vi "start panels.vi"(8 "error in":errorcluster) -> (0 "error out":errorcluster, 2 "vi names":string[](array[string]), 3 "vi refs":refnum<vi>[](array[refnum]))   [LabVIEW 2017]
panel:
  in  "visible":bool[](array[boolean])=[FALSE, FALSE, FALSE, FALSE, FALSE]
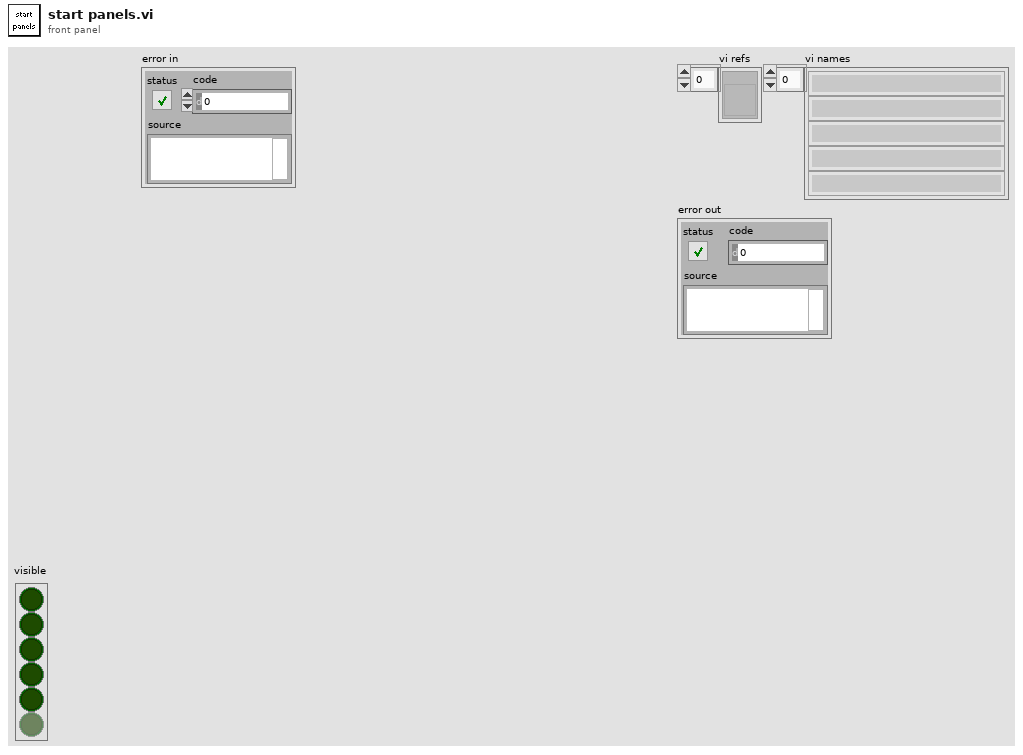
[diagram p1: front panel]
types:
  T1 = enum32{"Invalid", "Standard", "Closed", "Hidden", "Minimized", "Maximized"}
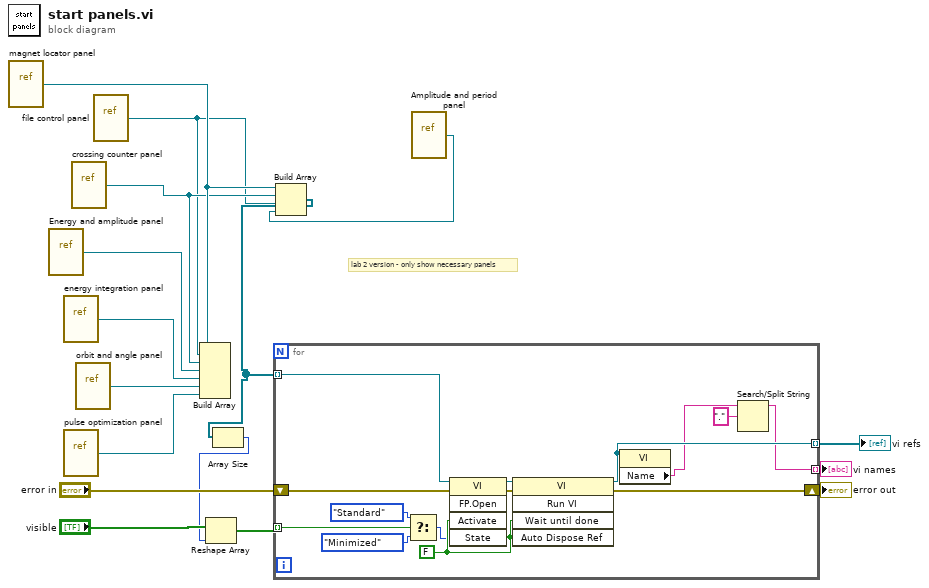
[diagram p0: block diagram]
diagram:
  # "lab 2 version - only show necessary panels"
  n1 = vi-ref "magnet locator panel.vi"() -> (w6:refnum<vi>)
  n2 = vi-ref "Energy and amplitude panel.vi"() -> (w15:refnum<vi>)
  n3 = vi-ref "energy integration panel.vi"() -> (w10:refnum<vi>)
  n4 = vi-ref "pulse optimization panel.vi"() -> (w14:refnum<vi>)
  n5 = vi-ref "crossing counter panel.vi"() -> (w5:refnum<vi>)
  n6 = vi-ref "orbit and angle panel.vi"() -> (w2:refnum<vi>)
  n7 = vi-ref "file control panel.vi"() -> (w3:refnum<vi>)
  n8 = Build Array(w6, w3, w5, w15, w10, w2, w14) -> ()  [unwired: 1 out]
  n9 = vi-ref "Amplitude and period panel.vi"() -> (w1:refnum<vi>)
  n10 = Build Array(w6, w5, w3, w1) -> (w4:refnum<vi>[])
  n11 = Array Size(array=w4) -> (size(s)=w7:i32)
  n12 = Reshape Array("visible", w7) -> (w8:bool[])
  n13 = for {
    tunnel: w4 -> [w30] mode=indexing
    tunnel: [w24] -> w13 mode=indexing
    shift-right: [w27] -> w11
    shift-left: "error in" -> [w26]
    tunnel: [w17] -> w12 mode=indexing
    tunnel: w8 -> [w21] mode=indexing
    w25 = FALSE ("Wait Until Done")
    n14 = Select(t=T1."Standard" ("Front Panel Window:State"), s=w21, f=T1."Minimized") -> (s? t:f=w20:T1)
    n15 = invoke class="VI" method="FP.Open"(reference=w30, error in=w26, "Activate"=w25, "State"=w20) -> (reference out=w29:refnum<vi>, error out=w28:errorcluster)  [unwired: 1 in, 3 out]
    n16 = invoke class="VI" method="Run VI"(reference=w29, error in=w28, "Wait until done"=w25, "Auto Dispose Ref"=w25) -> (reference out=w24:refnum<vi>, error out=w27:errorcluster)  [unwired: 1 in, 3 out]
    n17 = property class="VI"(reference=w24) -> ("Name"=w19:string)  [unwired: 1 in, 2 out]
    n18 = Search/Split String(string=w19, search string/char (-)=".") -> (substring before match=w17:string)  [unwired: 1 in, 2 out]
  }
  "vi refs" <- w13
  "vi names" <- w12
  "error out" <- w11
